vi "sutter driver 2.vi"(0 "VISA resource name":refnum<visa-resource-name>) -> ()   [LabVIEW 2016]
uses:
  <vilib>/Instr/_visa.llb/VISA Configure Serial Port (Instr).vi
panel:
  out "Numeric":i32
  in  "stop":bool
  out "error out":errorcluster
  out "Send Position":dbl[](array[numeric])
  out "Curent Position":dbl[](array[numeric])
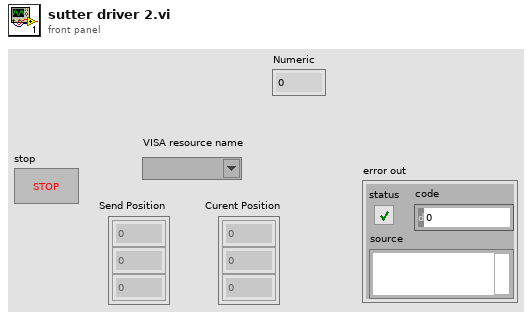
[diagram p1: front panel]
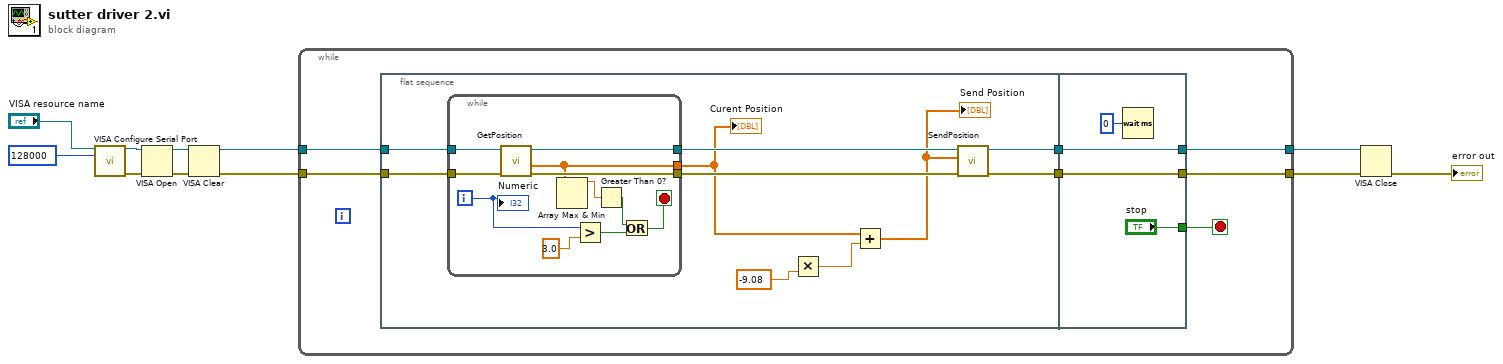
[diagram p0: block diagram]
diagram:
  n1 = call-poly "VISA Configure Serial Port"("VISA resource name"="VISA resource name", "baud rate (9600)"=u32 128000) -> ("VISA resource name out"=w9:refnum<visa-resource-name>, "error out"=w8:errorcluster)  [unwired: 12 in]
  n2 = VISA Open(error in (no error)=w8, VISA resource name=w9) -> (VISA resource name=w4:refnum<visa-resource-name>, error out=w3:errorcluster)  [unwired: 3 in]
  n3 = VISA Clear(VISA resource name=w4, error in (no error)=w3) -> (VISA resource name out=w2:refnum<visa-resource-name>, error out=w1:errorcluster)
  n4 = while {
    tunnel: w1 -> [w16]
    tunnel: [w17] -> w6
    tunnel: w2 -> [w15]
    tunnel: [w18] -> w7
    stop <- w12 stop-if-true
    n5 = flat-sequence {
      tunnel: w16 -> [w23]
      tunnel: w15 -> [w26]
      tunnel: [w28] -> w14
      tunnel: [w27] -> w13
      tunnel: [w42] -> w17
      tunnel: [w43] -> w18
      tunnel: w14 -> [w43]
      tunnel: w13 -> [w42]
      tunnel: ["stop"] -> w12
      frame #0 {
        n6 = while {
          tunnel: [w35] -> w19
          tunnel: w26 -> [w38]
          tunnel: [w37] -> w25
          tunnel: w23 -> [w39]
          tunnel: [w36] -> w24
          i -> [w33]
          stop <- w30 stop-if-true
          n7 = call "GetPosition.vi"("error in"=w39, "VISA resource name in"=w38) -> ("error out"=w36:errorcluster, "Position XYZ"=w35:dbl[], "VISA resource name out"=w37:refnum<visa-resource-name>)  [unwired: 3 in, 1 out]
          n8 = Array Max & Min(array=w35) -> (max value=w29:dbl)  [unwired: 3 out]
          n9 = Greater?(x=w33, y=3.0) -> (0:w32:bool)
          n10 = Greater Than 0?(x=w29) -> (x > 0?=w31:bool)
          n11 = Or(x=w31, y=w32) -> (x .or. y?=w30:bool)
          "Numeric" <- w33
        }
        "Curent Position" <- w19
        n12 = Multiply(y=-9.08 ("number: 0 to 1")) -> (x*y=w21:dbl)  [unwired: 1 in]
        n13 = Add(x=w19, y=w21) -> (x+y=w20:dbl[])
        "Send Position" <- w20
        n14 = call "SendPosition.vi"("error in"=w24, "Motor Position"=w20, "VISA resource In"=w25) -> ("error out"=w27:errorcluster, "VISA resource name out"=w28:refnum<visa-resource-name>)  [unwired: 5 in]
      }
      frame #1 {
        n15 = Wait (ms)(milliseconds to wait=u32 0) -> ()  [unwired: 1 out]
      }
    }
  }
  n16 = VISA Close(VISA resource name=w7, error in (no error)=w6) -> (error out=→"error out":errorcluster)
